vi "get_colormap.vi"(0 "Input Port in":T1 items=["Port 1", "Port 2", "Port 3", "Port 4"], 1 "Device Address":u8=2) -> (4 "Error":bool, 5 "Input Port out":T1 items=["Port 1", "Port 2", "Port 3", "Port 4"], 6 "length":i32, 7 "string":string, 8 "Status":string)   [LabVIEW 2016]
uses:
  <vilib>/NXT/Block Support/NXT_InputPort.ctl
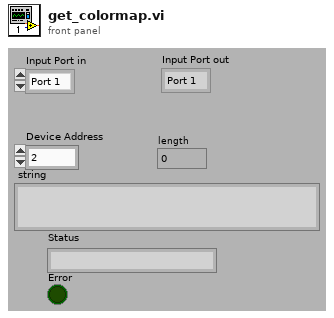
[diagram p1: front panel]
types:
  T1 = typedef "NXT_InputPort.ctl" = u32
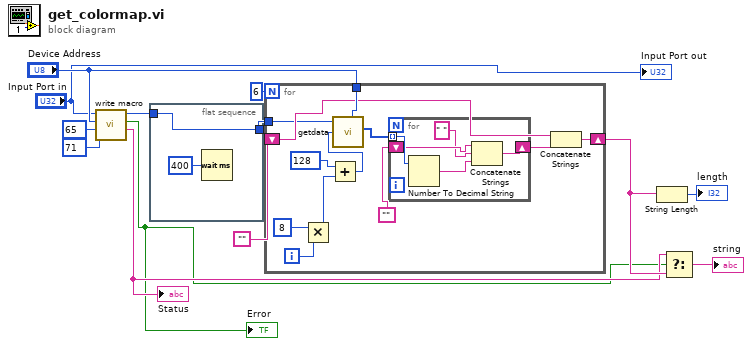
[diagram p0: block diagram]
diagram:
  n1 = call "write macro.vi"("Data byte"=u8 71, "Reg Address"=u8 65, "Address"="Device Address", "Input Port in"="Input Port in") -> ("Status"=w3:string, "Error"=w1:bool, "Input Port out"=w8:T1)  [unwired: 5 in]
  "Status" <- w3
  "Error" <- w1
  n2 = flat-sequence {
    tunnel: [w15] -> w9
    tunnel: w8 -> [w15]
    frame #0 {
      n3 = Wait (ms)(milliseconds to wait=u32 400) -> ()  [unwired: 1 out]
    }
  }
  n4 = for {
    N: 6 -> [_]
    tunnel: "Device Address" -> [w27]
    shift-right: [w24] -> w4
    shift-left: "" -> [w23]
    tunnel: w9 -> [w16]
    i -> [w20]
    n5 = Multiply(x=8, y=w20) -> (x*y=w19:i32)
    n6 = Add(x=128, y=w19) -> (x+y=w25:i32)
    n7 = call "getdata.vi"("Device Address"=w27, "Input Port in"=w16, "Reg Address"=w25) -> ("data"=w22:u8[])  [unwired: 2 in, 2 out]
    n8 = for {
      tunnel: w22 -> [w32] mode=indexing
      shift-right: [w31] -> w21
      shift-left: "" -> [w30]
      n9 = Number To Decimal String(number=w32) -> (decimal integer string=w29:string)  [unwired: 1 in]
      n10 = Concatenate Strings(w30, " " ("string"), w29) -> (w31:string)
    }
    n11 = Concatenate Strings(w23, w21) -> (w24:string)
  }
  n12 = String Length(string=w4) -> (length=→"length":i32)
  n13 = Select(t=w3, s=w1, f=w4) -> (s? t:f=→"string":string)
  "Input Port out" <- "Input Port in"
